vi "Write.vi"(8 "error in (no error)":errorcluster, 10 "Boolean":bool, 11 "Boolean in":refnum<class "OnChange_Boolean.lvclass">) -> (0 "error out":errorcluster, 3 "Boolean out":refnum<class "OnChange_Boolean.lvclass">)   [LabVIEW 2021, in "OnChange_Boolean.lvclass"]
doc: "Abstract Data Classes 2.1.1.13\nTim Streeter - TSA\nCopyright (c) 2025, TSA"
uses:
  OnChange_Boolean.lvclass
  OnChange_Boolean.lvclass/OnChange_Boolean.ctl
  <vilib>/TSA/Abstract Data Classes/Abs_Types/Boolean/Abs_Boolean.lvclass
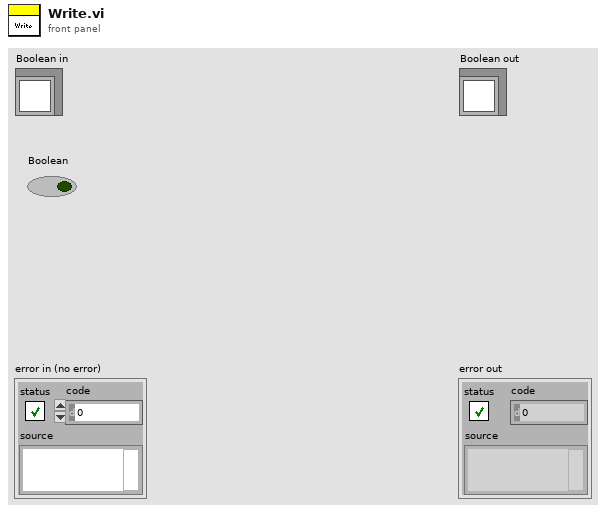
[diagram p1: front panel]
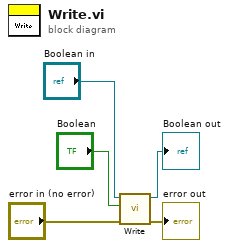
[diagram p0: block diagram]
diagram:
  n1 = call-parent "Write.vi"("error in (no error)"="error in (no error)", "Boolean"="Boolean", "Boolean in"="Boolean in") -> ("error out"=→"error out":errorcluster, "Boolean out"=→"Boolean out":refnum<class "OnChange_Boolean.lvclass">)  [unwired: 7 in]
